vi "Cleanup.vi"(8 "error in (no error)":errorcluster, 11 "Async Authorization in":refnum<class "Async Authorization.lvclass">) -> (0 "error out":errorcluster)   [LabVIEW 2020, in "OAuth2.lvlib" / "Async Authorization.lvclass"]
uses:
  Async Authorization.lvclass
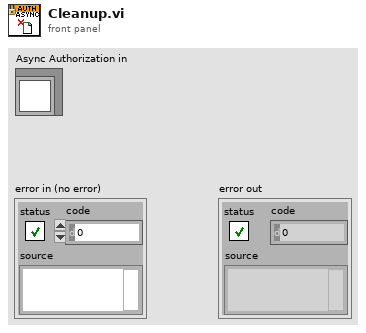
[diagram p1: front panel]
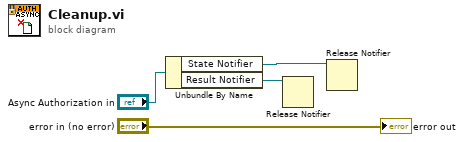
[diagram p0: block diagram]
diagram:
  n1 = Unbundle By Name("Async Authorization in") -> ("State Notifier"=w1:refnum<notifier>, "Result Notifier"=w2:refnum<notifier>)
  n2 = Release Notifier(notifier=w2) -> ()  [unwired: 2 in, 3 out]
  n3 = Release Notifier(notifier=w1) -> ()  [unwired: 2 in, 3 out]
  "error out" <- "error in (no error)"
